vi "dfd_Sort Poles.vi"(1 "poles":cdb[](array[numeric])) -> (0 "sorted poles":cdb[](array[numeric]))   [LabVIEW 2017, in "NI_DigFilterLicensed.lvlib"]
uses:
  <vilib>/addons/Digital Filter Design/NI_DigFilterLicensed.lvlib
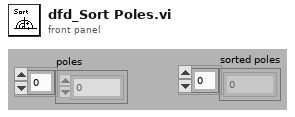
[diagram p1: front panel]
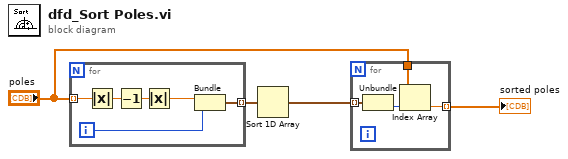
[diagram p0: block diagram]
diagram:
  n1 = for {
    tunnel: "poles" -> [w10] mode=indexing
    tunnel: [w7] -> w2 mode=indexing
    i -> [w8]
    n2 = Absolute Value(x=w10) -> (abs(x)=w9:dbl)
    n3 = Decrement(x=w9) -> (x-1=w6:dbl)
    n4 = Absolute Value(x=w6) -> (abs(x)=w5:dbl)
    n5 = Bundle(w5, w8) -> (w7:cluster{dbl, i32})  [unwired: 1 out]
  }
  n6 = Sort 1D Array(array=w2) -> (sorted array=w1:cluster{dbl, i32}[])
  n7 = for {
    tunnel: "poles" -> [w14]
    tunnel: w1 -> [w13] mode=indexing
    tunnel: [w11] -> w4 mode=indexing
    n8 = Unbundle(w13) -> (w12:i32)  [unwired: 1 out]
    n9 = Index Array(array=w14, index=w12) -> (element=w11:cdb)
  }
  "sorted poles" <- w4
